vi "Dark Current Test (Brute Force Version).vi"() -> ()   [LabVIEW 2020]
uses:
  <vilib>/DAQmx/create/channels.llb/DAQmx Create Channel (DO-Digital Output).vi
panel:
  out "Test Is Running (Red)\nTest Is Stopped (Green)":bool
  in  "Start":bool
  out "Failed Tubes":string[](array[string])
  in  "Barcodes in 4":string[](array[string])
  in  "Barcodes in 3":string[](array[string])
  in  "Barcodes in 2":string[](array[string])
  in  "Barcodes in":string[](array[string])
  out "Actual Voltage Level (V)":dbl format="%#_13g"
  out "Power Supply Trip":bool
  out "Actual Current Limit (nA)":dbl format="%#_13g"
  out "Mesurnment Itteration":i32
  in  "stop":bool
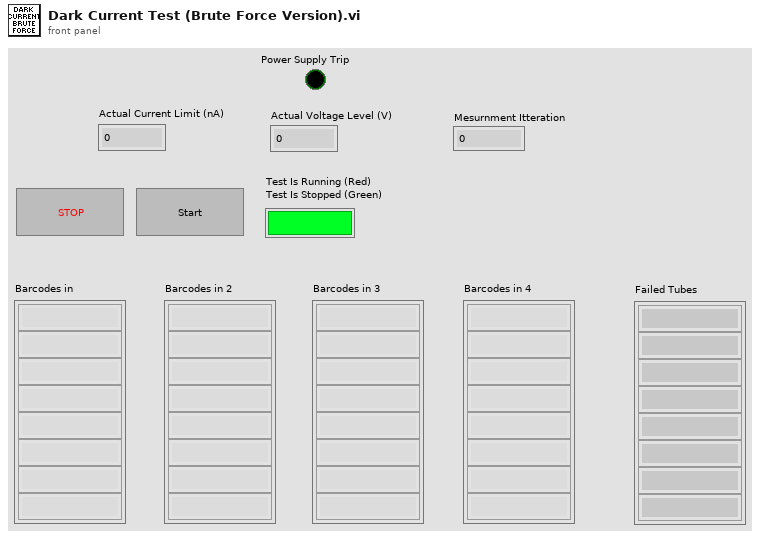
[diagram p1: front panel]
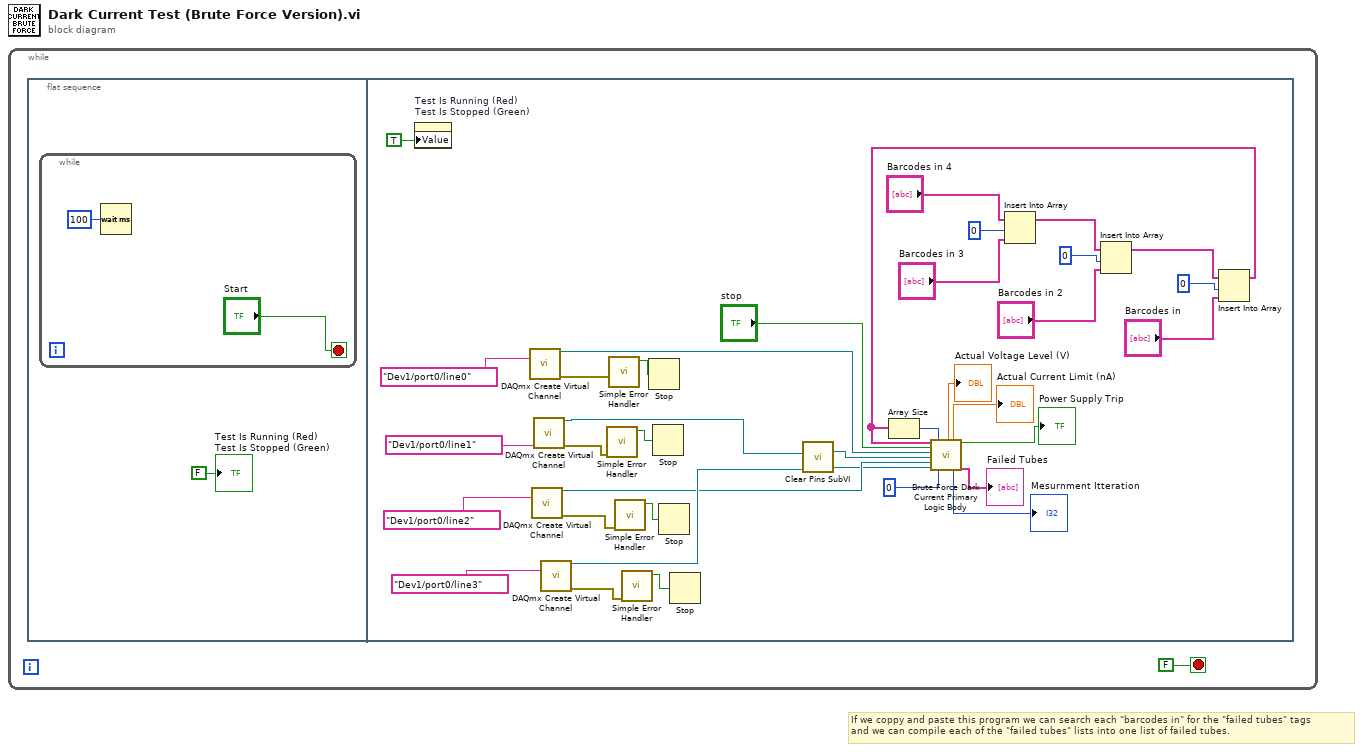
[diagram p0: block diagram]
diagram:
  # "If we coppy and paste this program we can search each \"barcodes in\" for the \"failed tubes\" tags\nand we can compile each of the \"failed tubes\" lists into one list of failed tubes."
  n1 = while {
    stop <- FALSE stop-if-true
    n2 = flat-sequence {
      frame #0 {
        n3 = while {
          stop <- "Start" stop-if-true
          n4 = Wait (ms)(milliseconds to wait=u32 100) -> ()  [unwired: 1 out]
        }
        "Test Is Running (Red)\nTest Is Stopped (Green)" <- FALSE ("Start LED")
      }
      frame #1 {
        n5 = property on="Test Is Running (Red)\nTest Is Stopped (Green)" class="Bool (strict)"("Value"=TRUE) -> ()  [unwired: 2 in, 2 out]
        n6 = call-poly <vilib>:"DAQmx Create Virtual Channel.vi"("lines"=tag "Dev1/port0/line0" ("Data Pin")) -> ("task out"=w17:refnum<k21>, "error out"=w37:errorcluster)  [unwired: 13 in]
        n7 = call-poly <vilib>:"DAQmx Create Virtual Channel.vi"("lines"=tag "Dev1/port0/line2" ("Write Pin")) -> ("task out"=w15:refnum<k21>, "error out"=w35:errorcluster)  [unwired: 13 in]
        n8 = call-poly <vilib>:"DAQmx Create Virtual Channel.vi"("lines"=tag "Dev1/port0/line1" ("Sync Pin")) -> ("task out"=w29:refnum<k21>, "error out"=w36:errorcluster)  [unwired: 13 in]
        n9 = call-poly <vilib>:"DAQmx Create Virtual Channel.vi"("lines"=tag "Dev1/port0/line3" ("Clear Pin")) -> ("task out"=w28:refnum<k21>, "error out"=w34:errorcluster)  [unwired: 13 in]
        n10 = call <vilib>:"Simple Error Handler.vi"("error in (no error)"=w36) -> ("error?"=w30:bool)  [unwired: 4 in, 4 out]
        n11 = call <vilib>:"Simple Error Handler.vi"("error in (no error)"=w37) -> ("error?"=w33:bool)  [unwired: 4 in, 4 out]
        n12 = call <vilib>:"Simple Error Handler.vi"("error in (no error)"=w35) -> ("error?"=w31:bool)  [unwired: 4 in, 4 out]
        n13 = call <vilib>:"Simple Error Handler.vi"("error in (no error)"=w34) -> ("error?"=w32:bool)  [unwired: 4 in, 4 out]
        n14 = Stop(stop? (T)=w33) -> ()
        n15 = Stop(stop? (T)=w30) -> ()
        n16 = Stop(stop? (T)=w31) -> ()
        n17 = Stop(stop? (T)=w32) -> ()
        n18 = call "Clear Pins SubVI.vi"("Clear Pin Task In"=w28, "Sync Pin Task In"=w29) -> ("Clear Pin Task Out"=w14:refnum<k21>, "Sync Pin Task Out"=w16:refnum<k21>)  [unwired: 8 in]
        n19 = Insert Into Array(array="Barcodes in 4", index=0, new element="Barcodes in 3") -> (w23:string[])
        n20 = Insert Into Array(array=w23, index=0, new element="Barcodes in 2") -> (w19:string[])
        n21 = Insert Into Array(array=w19, index=0, new element="Barcodes in") -> (w13:string[])
        n22 = Array Size(array=w13) -> (size(s)=w11:i32)
        n23 = call "Brute Force Dark Current Primary Logic Body.vi"("Barcodes in"=w13, "stop"="stop", "Data Pin in"=w17, "Sync Pin in"=w16, "Write Pin in"=w15, "Clear Pin in"=w14, "Number of Tubes"=w11, "Channel #"=0) -> ("Actual Voltage Level (V)"=→"Actual Voltage Level (V)":dbl, "Actual Current Limit (nA)"=→"Actual Current Limit (nA)":dbl, "Mesurnment Itteration"=→"Mesurnment Itteration":i32, "Power Supply Trip"=→"Power Supply Trip":bool, "Failed Tubes"=→"Failed Tubes":string[])  [unwired: 3 in, 4 out]
      }
    }
  }
